vi "EnsaioJigaAutomatizado.vi"() -> ()   [LabVIEW 2025]
uses:
  Estados_Ensaio.ctl
  <vilib>/DAQmx/create/channels.llb/DAQmx Create Channel (DO-Digital Output).vi
  <vilib>/DAQmx/write.llb/DAQmx Write (Digital 1D Bool 1Chan 1Samp).vi
  <vilib>/Utility/file.llb/Write Delimited Spreadsheet (DBL).vi
panel:
  out "Tempo Decorrido (Motor) (s) 2":dbl
  in  "Braco Resistor - 0.68//0.68 2":bool
  in  "Braco Resistor -  0.47//0.47 2":bool
  in  "Braco Resistor - 0.47 2":bool
  in  "Braco Resistor - 1 MOSFET 2":bool
  out "error out 2":errorcluster
  out "Motor  Desligado":i32
  out "Motor Ligado":i32
  in  "module path":path
  in  "Iniciar":bool
  out "Estado Atual":string
  in  "ABORTAR ENSAIO":bool
  out "Tempo Decorrido (Entre braços) (s)":dbl
  out "Tempo Decorrido (Pré-Carga) (s)":dbl
  out "Ativado Braço 7":bool
  out "Pré - Carga Braço 7":bool
  out "Ativado Braço 6":bool
  out "Pré - Carga Braço 6":bool
  out "Ativado Braço 5":bool
  out "Pré - Carga Braço 5":bool
  out "Ativado Braço 4":bool
  out "Pré - Carga Braço 4":bool
  out "Ativado Braço 3":bool
  out "Pré - Carga Braço 3":bool
  out "Ativado Braço  2":bool
  out "Pré - Carga Braço 2":bool
  out "Ativado Braço 1":bool
  out "Pré - Carga Braço 1":bool
  out "Ensaio Iniciado":bool
  in  "Parada while":bool
  in  "Tempo de desligamento entre braços (s)":dbl
  in  "Tempo de pré-carga (s)":dbl
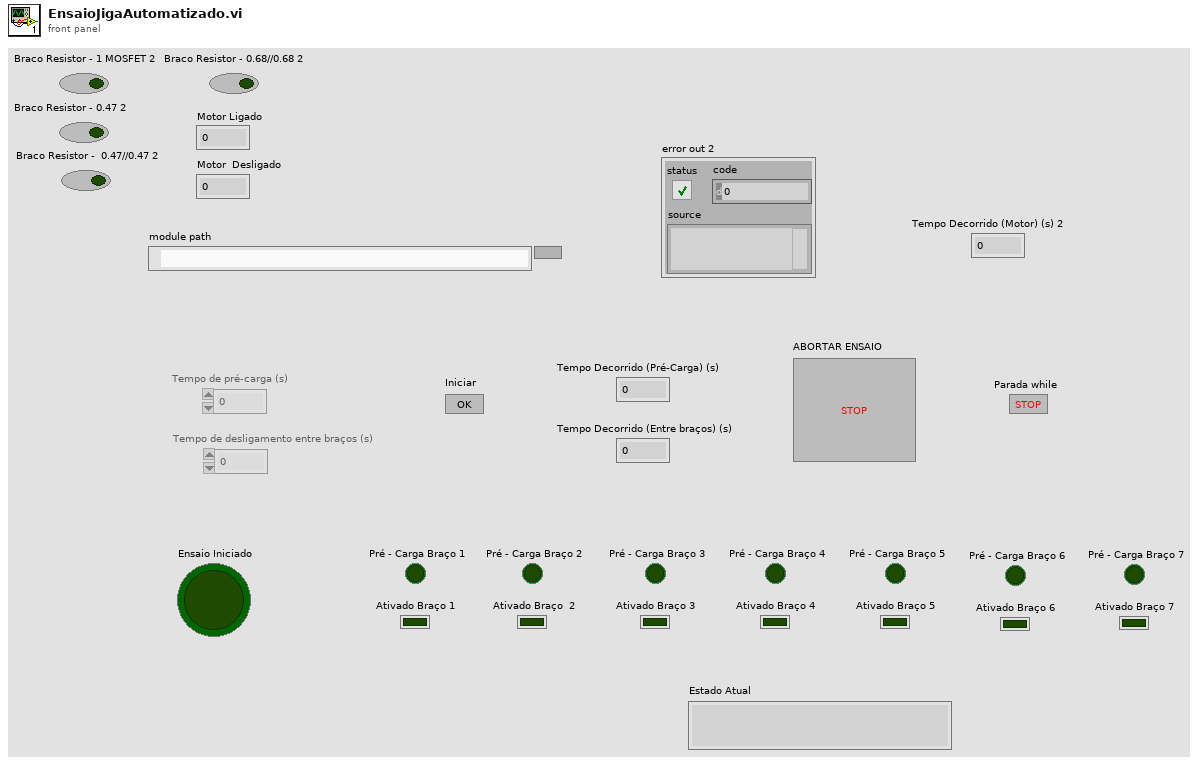
[diagram p1: front panel]
types:
  T1 = typedef "Estados_Ensaio.ctl" = enum16{"Idle", "AtivaPreCarga", "AguardaPreCarga", "AtivaBracosDesativaPreCarga", "DesativaBraco", "Fim", "Abortar", "AtivaBracos", "AguardaAtrasoPreCarga", "ComandoMotor"}
  T2 = enum8{"Enabled", "Disabled", "Disabled and Grayed Out"}
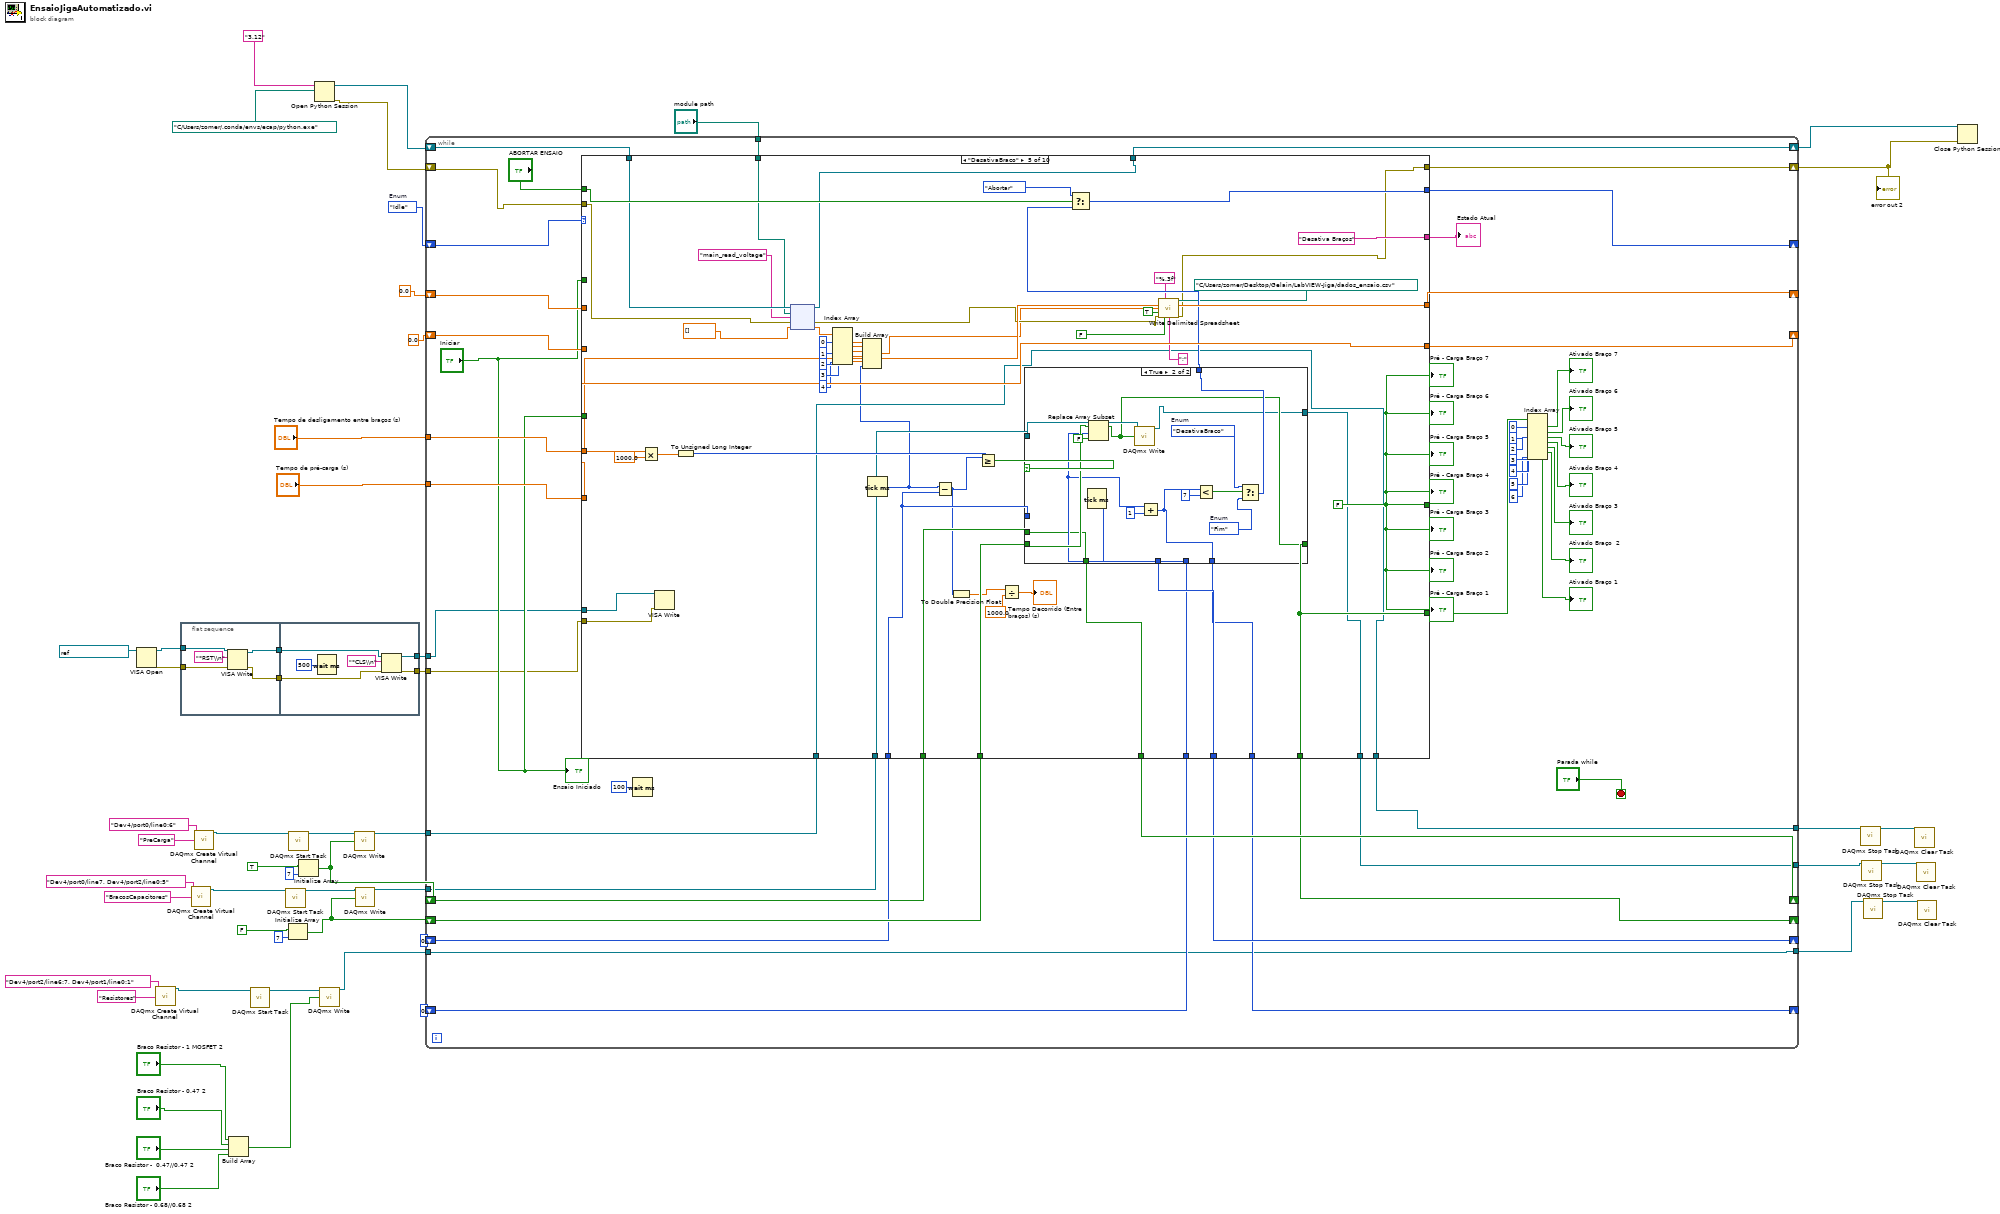
[diagram p0: block diagram]
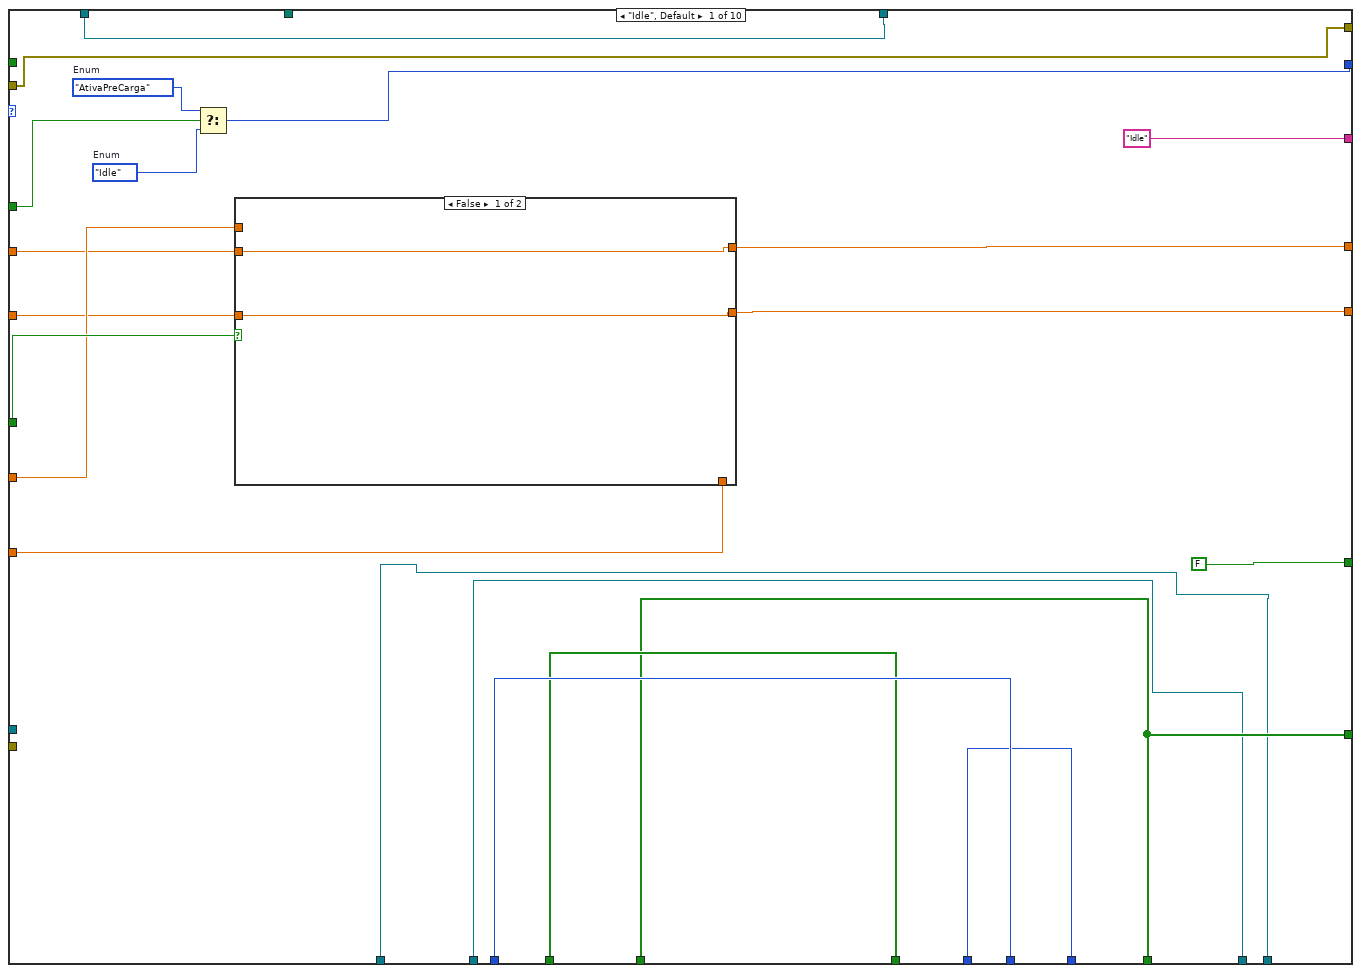
[diagram p2: hidden frame]
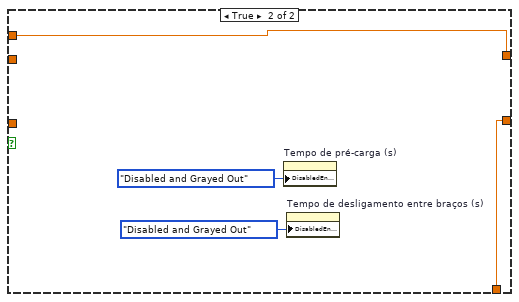
[diagram p3: hidden frame]
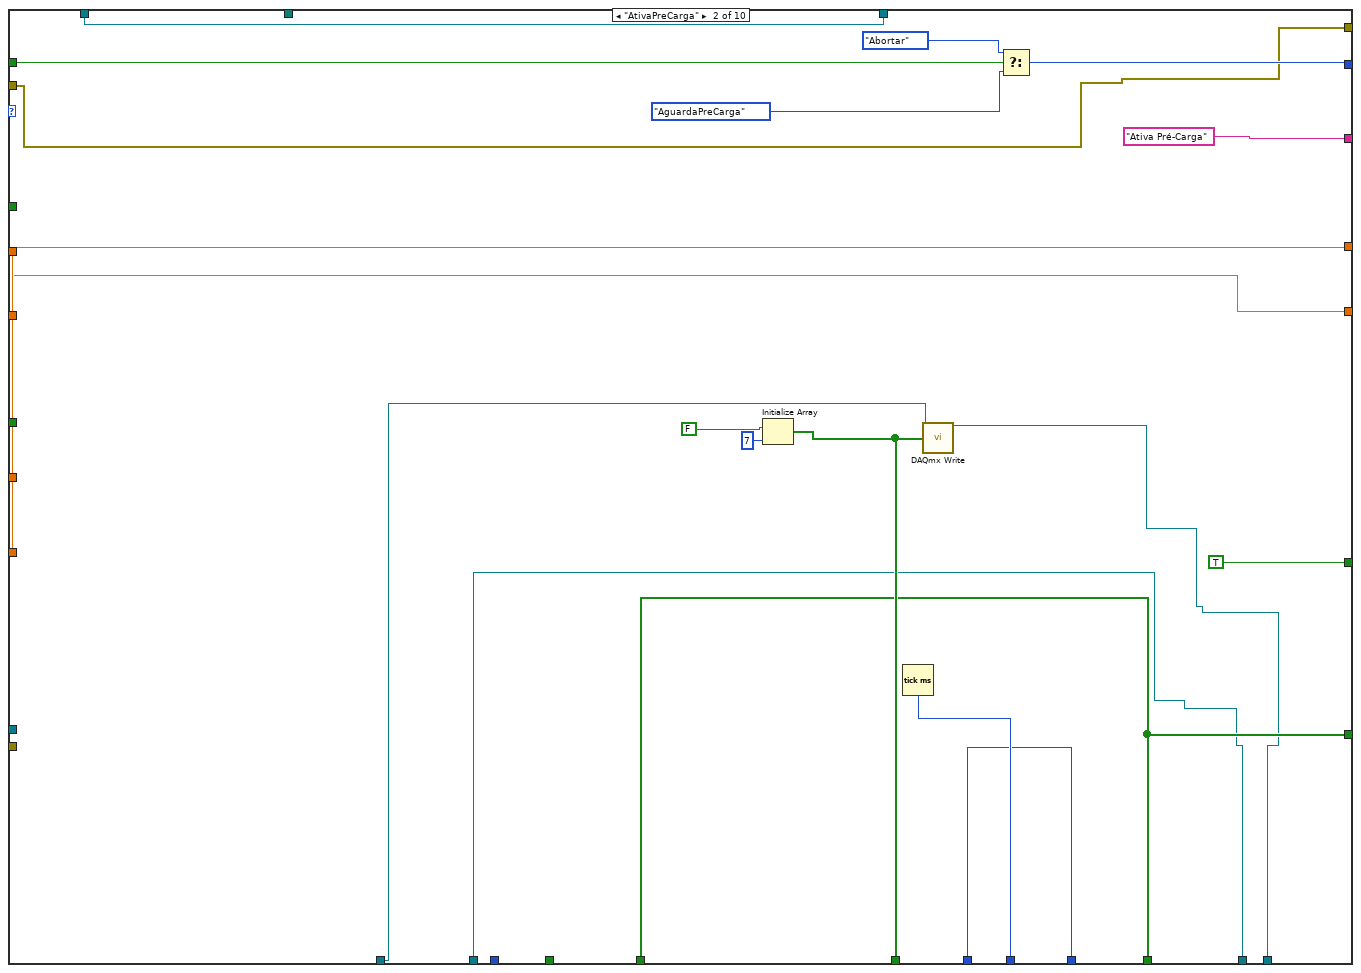
[diagram p4: hidden frame]
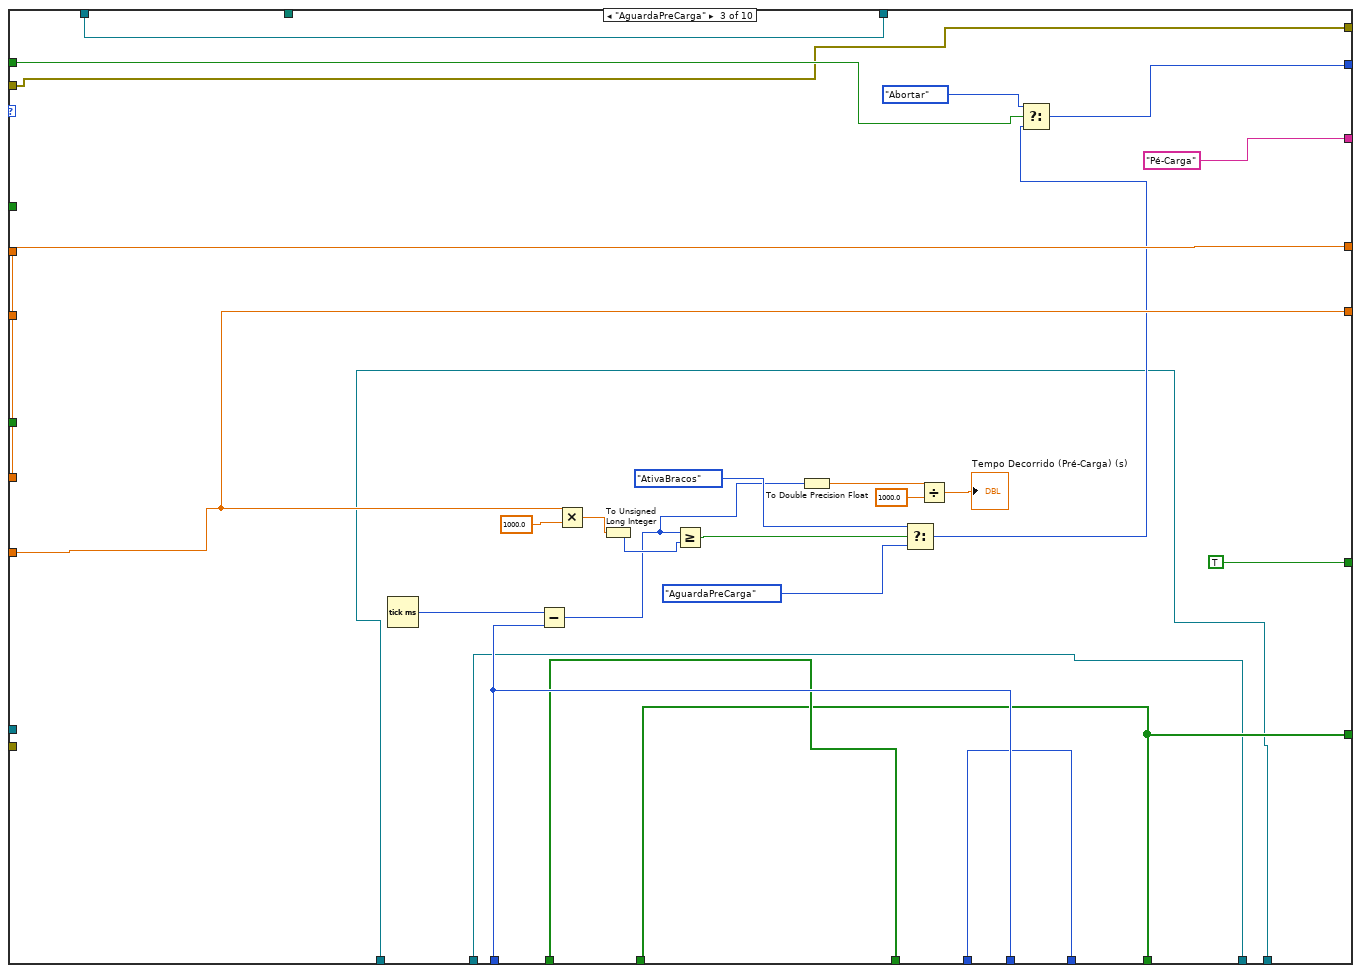
[diagram p5: hidden frame]
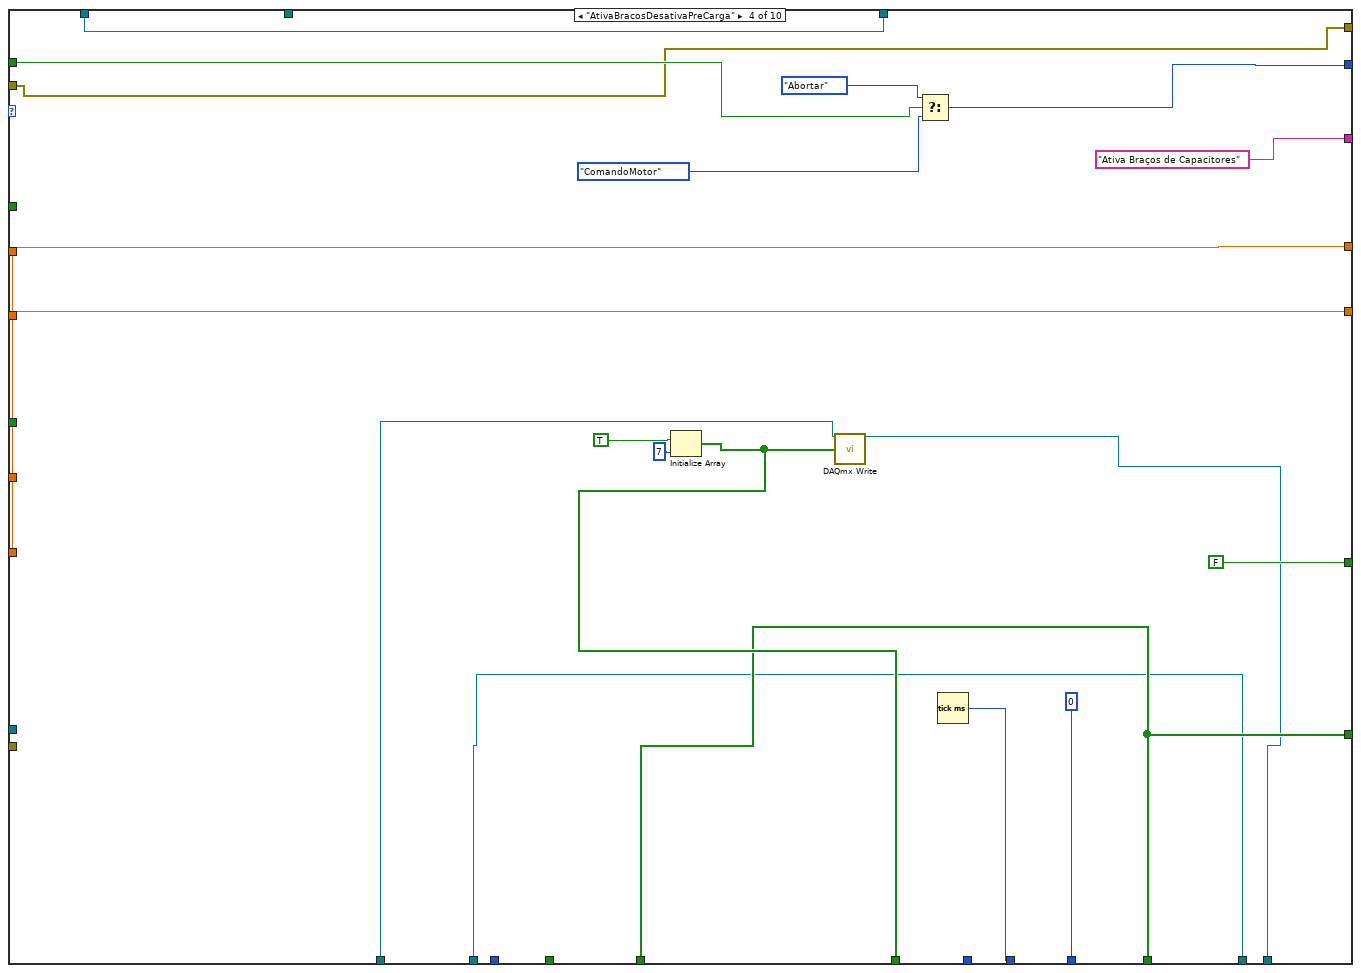
[diagram p6: hidden frame]
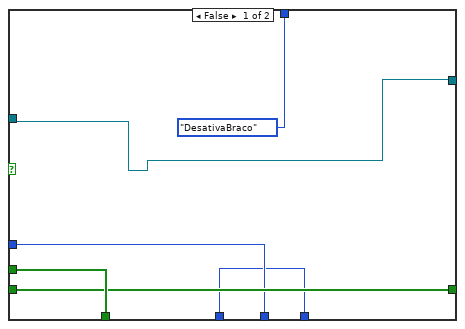
[diagram p7: hidden frame]
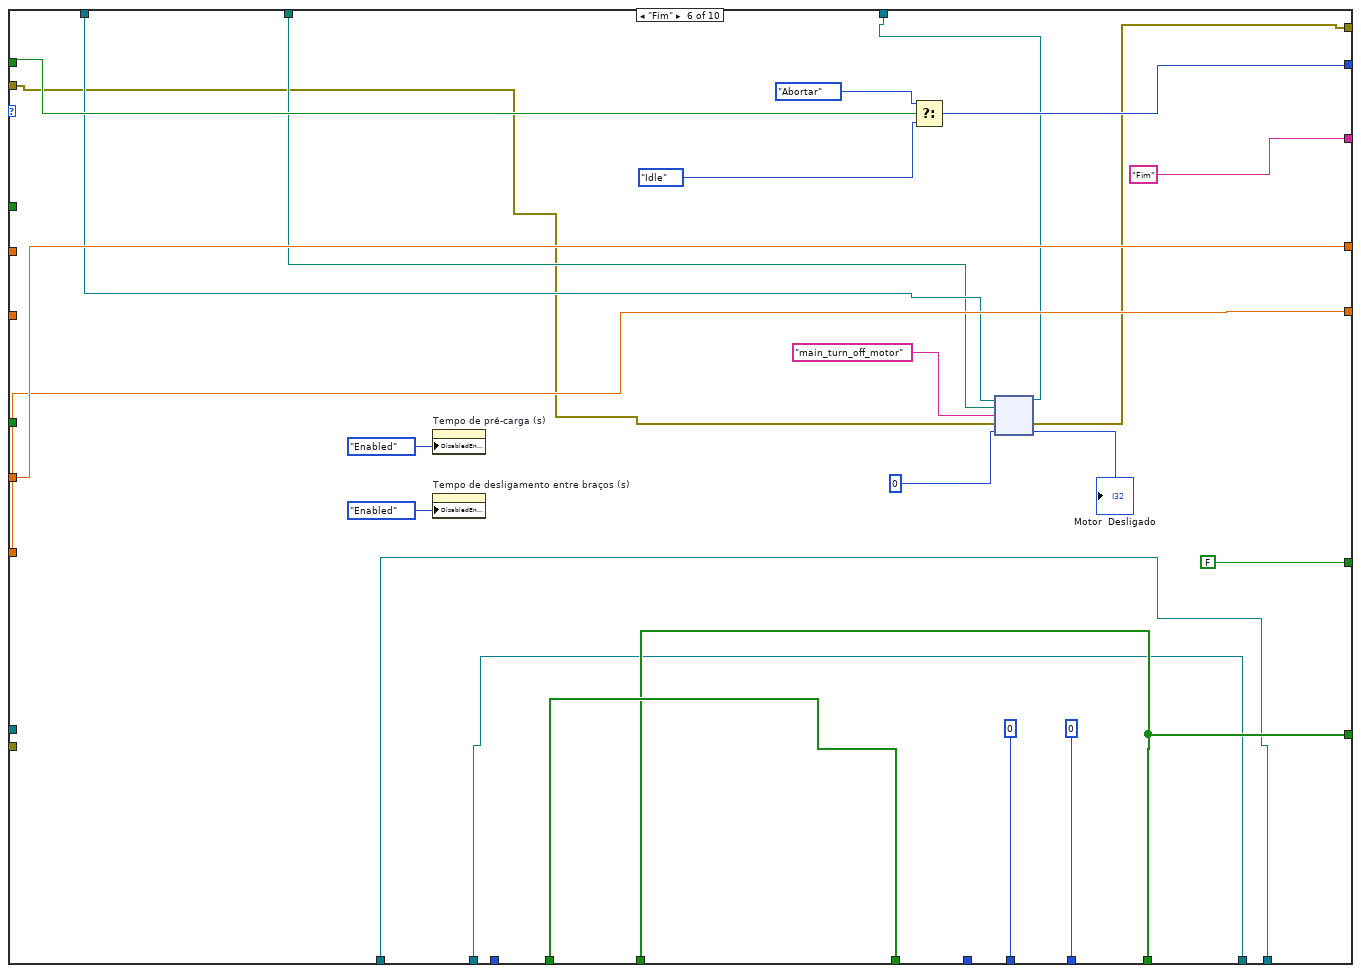
[diagram p8: hidden frame]
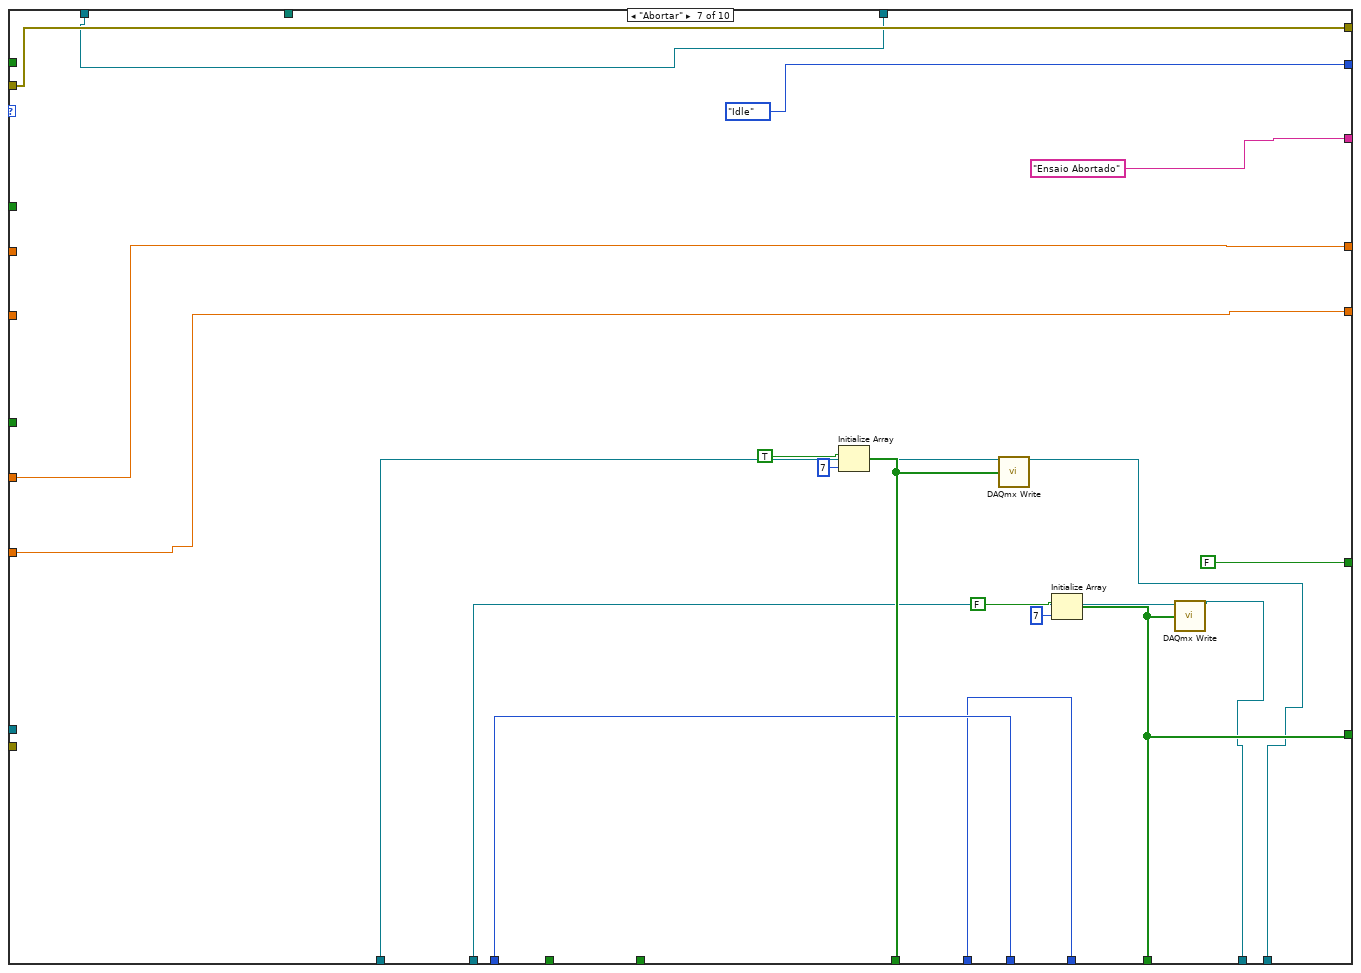
[diagram p9: hidden frame]
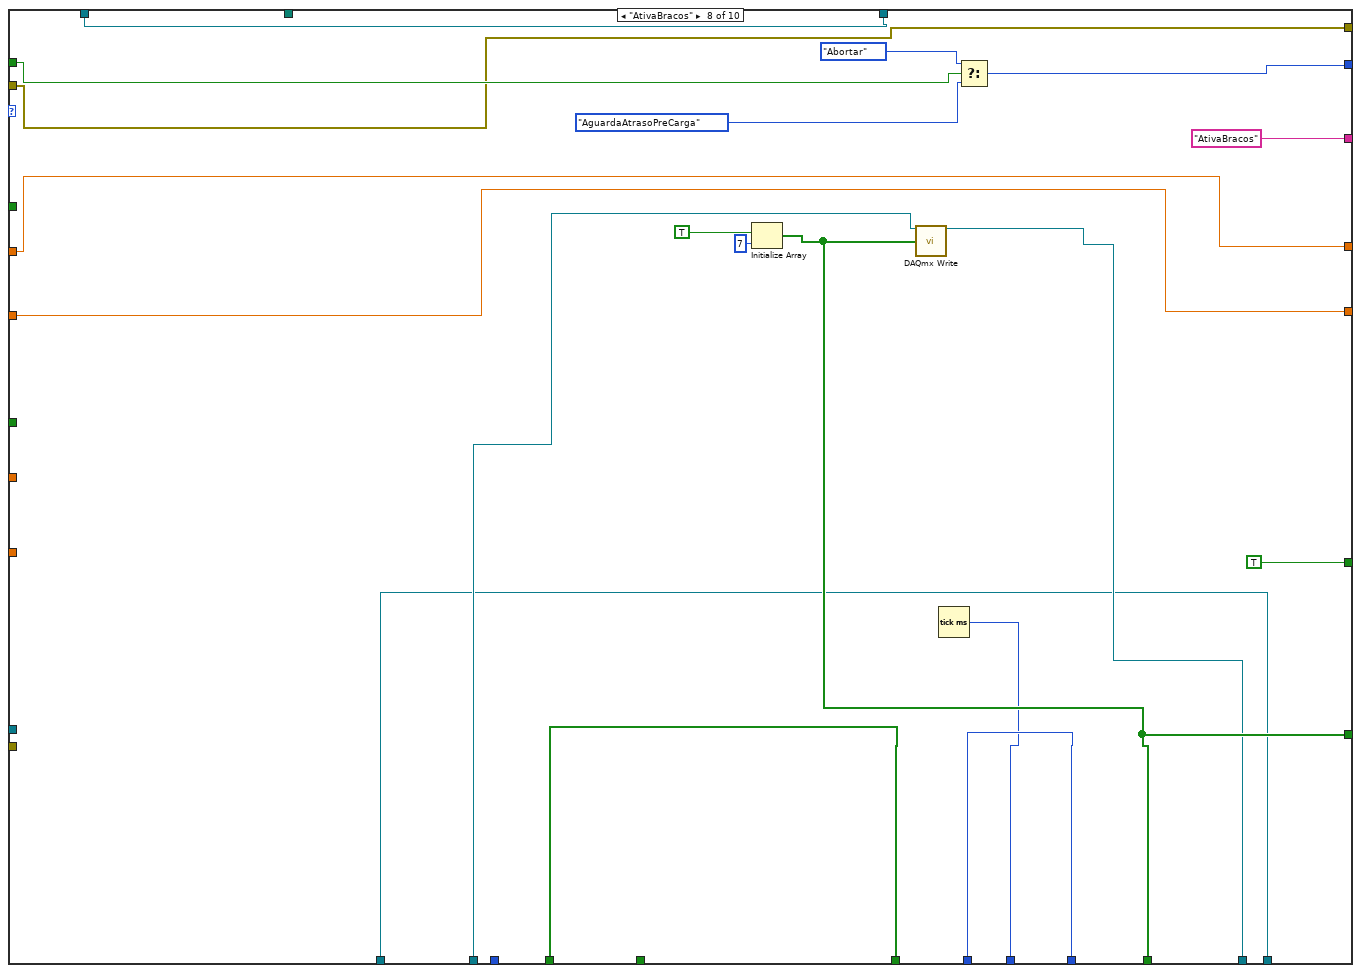
[diagram p10: hidden frame]
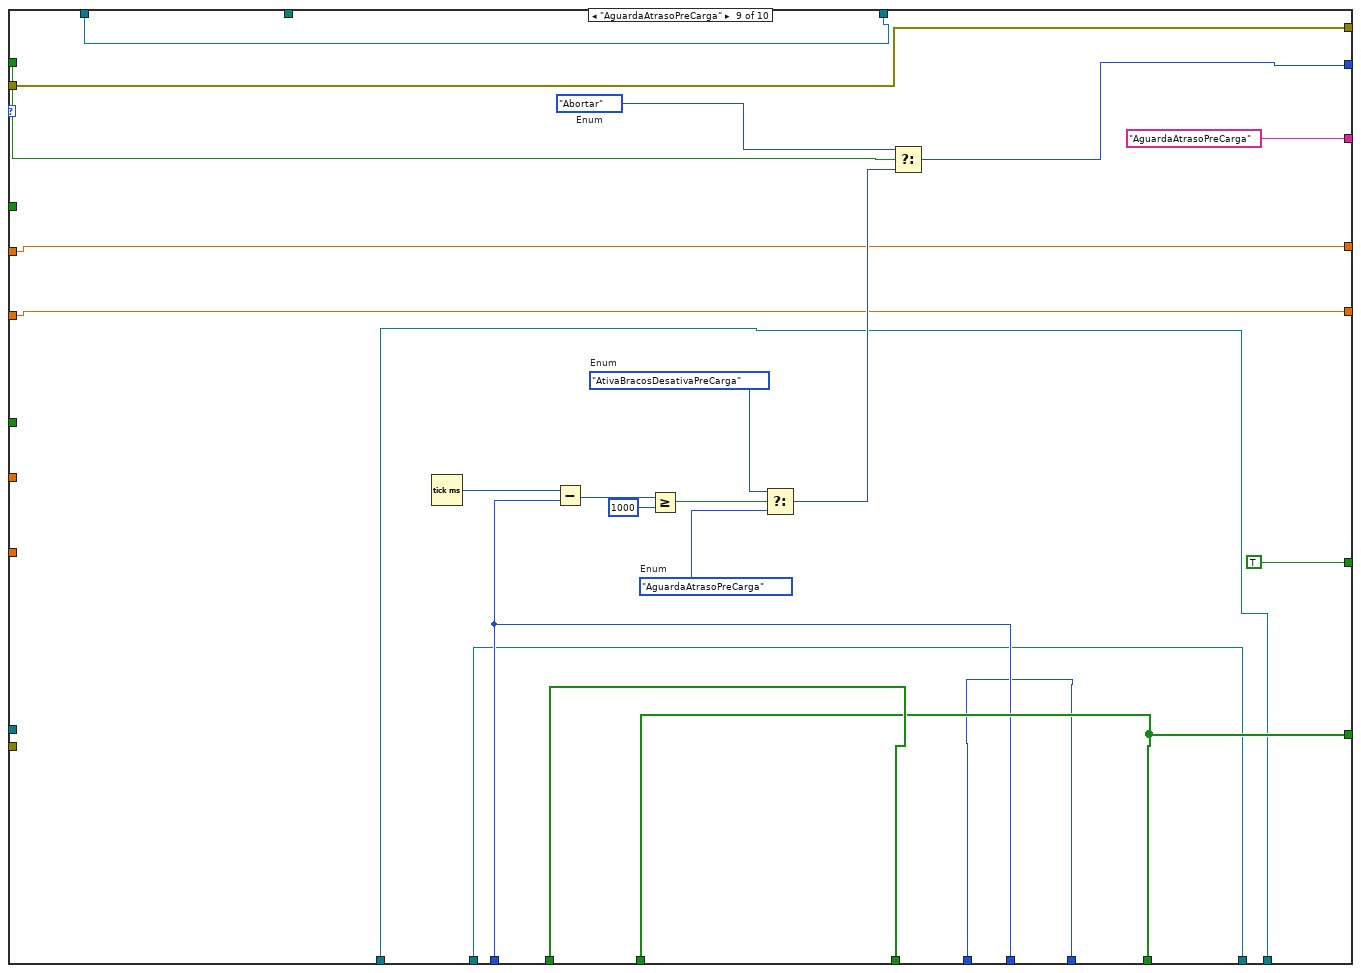
[diagram p11: hidden frame]
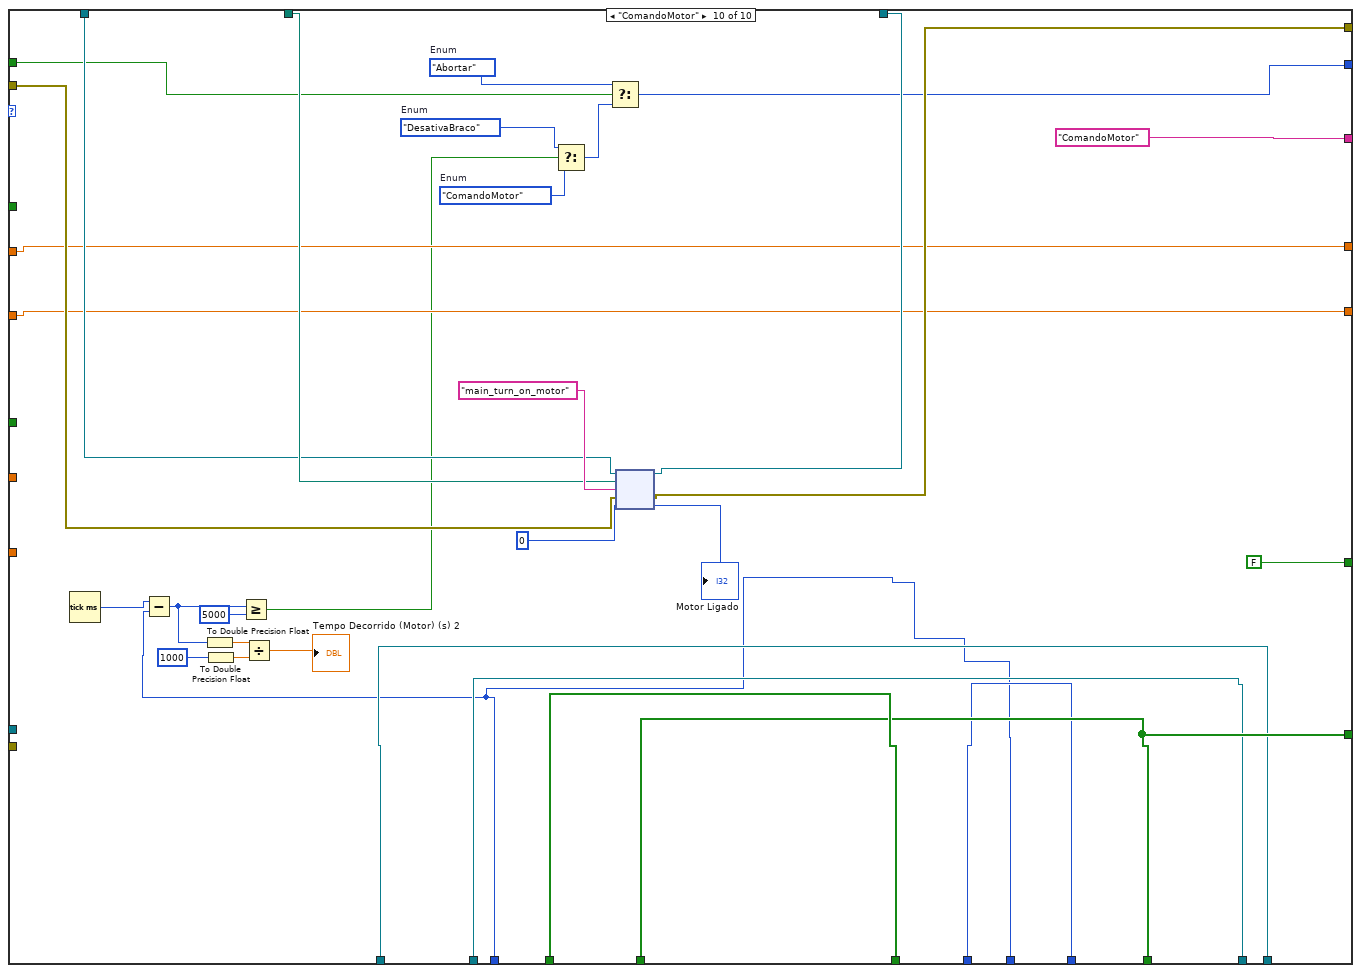
[diagram p12: hidden frame]
diagram:
  w51 = Estados_Ensaio."Idle"  # Enum
  n1 = VISA Open(VISA resource name=refnum<visa-resource-name> "GPIB0::1::INSTR") -> (VISA resource name=w6:refnum<visa-resource-name>, error out=w5:errorcluster)  [unwired: 4 in]
  n2 = call-poly <vilib>:"DAQmx Create Virtual Channel.vi"("lines"=tag "Dev4/port2/line6:7, Dev4/port1/line0:1", "name to assign"="Resistores") -> ("task out"=w17:refnum<k21>)  [unwired: 12 in, 1 out]
  n3 = flat-sequence {
    tunnel: w6 -> [w57]
    tunnel: w5 -> [w56]
    tunnel: [w55] -> w4
    tunnel: [w54] -> w3
    tunnel: w4 -> [w62]
    tunnel: w3 -> [w61]
    tunnel: [w60] -> w2
    tunnel: [w59] -> w1
    frame #0 {
      n4 = VISA Write(VISA resource name=w57, write buffer="*RST\\n", error in (no error)=w56) -> (VISA resource name out=w55:refnum<visa-resource-name>, error out=w54:errorcluster)  [unwired: 1 out]
    }
    frame #1 {
      n5 = Wait (ms)(milliseconds to wait=u32 500) -> ()  [unwired: 1 out]
      n6 = VISA Write(VISA resource name=w62, write buffer="*CLS\\n", error in (no error)=w61) -> (VISA resource name out=w60:refnum<visa-resource-name>, error out=w59:errorcluster)  [unwired: 1 out]
    }
  }
  n7 = call-poly <vilib>:"DAQmx Create Virtual Channel.vi"("lines"=tag "Dev4/port0/line7, Dev4/port2/line0:5", "name to assign"="BracosCapacitores") -> ("task out"=w43:refnum<k21>)  [unwired: 12 in, 1 out]
  n8 = call-poly <vilib>:"DAQmx Create Virtual Channel.vi"("lines"=tag "Dev4/port0/line0:6", "name to assign"="PreCarga") -> ("task out"=w46:refnum<k21>)  [unwired: 12 in, 1 out]
  n9 = Build Array("Braco Resistor - 1 MOSFET 2", "Braco Resistor - 0.47 2", "Braco Resistor -  0.47//0.47 2", "Braco Resistor - 0.68//0.68 2") -> (w11:bool[])
  n10 = call <vilib>:"DAQmx Start Task.vi"("task/channels in"=w17) -> ("task out"=w16:refnum<k21>)  [unwired: 13 in, 1 out]
  n11 = call <vilib>:"DAQmx Start Task.vi"("task/channels in"=w43) -> ("task out"=w39:refnum<k21>)  [unwired: 13 in, 1 out]
  n12 = Initialize Array(FALSE, 7 ("dimension size")) -> (w35:bool[])
  n13 = call <vilib>:"DAQmx Start Task.vi"("task/channels in"=w46) -> ("task out"=w42:refnum<k21>)  [unwired: 13 in, 1 out]
  n14 = Initialize Array(TRUE, 7 ("dimension size")) -> (w34:bool[])
  n15 = Open Python Session(python version="3.12" ("Python version"), python path=path "C:/Users/zomer/.conda/envs/ecap/python.exe" ("Python path")) -> (session out=w27:refnum<k35>, error out=w26:errorcluster)  [unwired: 1 in]
  n16 = call-poly <vilib>:"DAQmx Write.vi"("task/channels in"=w16, "data"=w11) -> ("task out"=w8:refnum<k21>)  [unwired: 11 in, 2 out]
  n17 = call-poly <vilib>:"DAQmx Write.vi"("task/channels in"=w42, "data"=w34) -> ("task out"=w36:refnum<k21>)  [unwired: 11 in, 2 out]
  n18 = call-poly <vilib>:"DAQmx Write.vi"("task/channels in"=w39, "data"=w35) -> ("task out"=w32:refnum<k21>)  [unwired: 11 in, 2 out]
  n19 = while {
    shift-right: [w112] -> _
    shift-left: 0.0 ("Tempo de desligamento entre braços (s)") -> [w107]
    shift-right: [w111] -> _
    shift-left: 0.0 ("Tempo de pré-carga (s)") -> [w106]
    shift-right: [w80] -> _
    shift-left: w51 -> [w79]
    tunnel: "Tempo de desligamento entre braços (s)" -> [w109]
    tunnel: "Tempo de pré-carga (s)" -> [w108]
    shift-right: [w105] -> _
    shift-left: w34 -> [w99]
    shift-right: [w103] -> _
    shift-left: w35 -> [w102]
    shift-right: [w101] -> _
    shift-left: u32 0 ("millisecond timer value") -> [w100]
    tunnel: w36 -> [w104]
    tunnel: w32 -> [w98]
    shift-right: [w97] -> _
    shift-left: 0 -> [w96]
    tunnel: "module path" -> [w75]
    shift-right: [w73] -> w25
    shift-left: w27 -> [w74]
    shift-right: [w71] -> w24
    shift-left: w26 -> [w72]
    tunnel: [w69] -> w23
    tunnel: [w68] -> w20
    tunnel: [w67] -> w9
    tunnel: w8 -> [w67]
    tunnel: w2 -> [w66]
    tunnel: w1 -> [w65]
    stop <- "Parada while" stop-if-true
    n20 = case shown="\"DesativaBraco\"" w79 {
      tunnel: [w130 w148 w167 w193 w237 w294 Estados_Ensaio."Idle" ("Enum") w330 w356 w376] -> w80
      tunnel: "Iniciar" -> [w131 _ _ _ _ _ _ _ _ _]
      tunnel: "Iniciar" -> [w134 _ _ _ _ _ _ _ _ _]
      tunnel: [w133 w154 w186 w205 w241 w305 w323 w336 w354 w386] -> w112
      tunnel: [w132 w153 w178 w204 w260 w304 w322 w335 w353 w385] -> w111
      tunnel: [w120 w151 w174 w191 w246 w297 w314 w340 w350 w382] -> w95
      tunnel: [FALSE ("Pré - Carga Braço 4") TRUE ("Pré - Carga Braço 4") TRUE ("Pré - Carga Braço 4") FALSE ("Pré - Carga Braço 4") FALSE ("Pré - Carga Braço 4") FALSE ("Pré - Carga Braço 4") FALSE ("Pré - Carga Braço 4") TRUE ("Pré - Carga Braço 4") TRUE ("Pré - Carga Braço 4") FALSE ("Pré - Carga Braço 4")] -> w110
      tunnel: w109 -> [w126 w154 w186 w205 w241 w305 w323 _ _ _]
      tunnel: w108 -> [w125 w153 w178 w204 w260 w304 w322 _ _ _]
      tunnel: w107 -> [w124 _ _ _ _ _ _ w336 w354 w386]
      tunnel: w106 -> [w123 _ _ _ _ _ _ w335 w353 w385]
      tunnel: [w121 w157 w177 w200 w255 w298 w318 w338 w351 w383] -> w105
      tunnel: w104 -> [w115 w156 w161 w199 w222 w283 w317 w325 w344 w379]
      tunnel: [w120 w151 w174 w191 w246 w297 w314 w340 w350 w382] -> w103
      tunnel: w102 -> [w120 w151 w174 w191 w248 w297 _ _ w350 w382]
      tunnel: [w122 w152 w179 w198 w253 u32 0 ("millisecond timer value") w312 w329 w349 w366] -> w101
      tunnel: w100 -> [w122 _ w179 _ w252 _ w312 _ w349 w366]
      tunnel: w99 -> [w121 _ w177 _ w254 w298 _ w338 w351 w383]
      tunnel: w98 -> [w114 w141 w160 w187 w249 w282 w313 w341 w345 w380]
      tunnel: [w119 w150 w173 0 w251 0 w311 w337 w348 w381] -> w97
      tunnel: w96 -> [w119 w150 w173 _ w250 _ w311 w337 w348 w381]
      tunnel: "ABORTAR ENSAIO" -> [_ w147 w165 w194 w238 w293 _ w331 w358 w388]
      tunnel: ["Idle" "Ativa Pré-Carga" "Pé-Carga" "Ativa Braços de Capacitores" "Desativa Braços" "Fim" "Ensaio Abortado" "AtivaBracos" "AguardaAtrasoPreCarga" "ComandoMotor"] -> w77
      tunnel: w75 -> [_ _ _ _ w233 w287 _ _ _ w393]
      tunnel: w74 -> [w117 w144 w163 w190 w235 w288 w308 w328 w347 w392]
      tunnel: [w117 w144 w163 w190 w232 w285 w308 w328 w347 w391] -> w73
      tunnel: w72 -> [w116 w143 w162 w189 w231 w286 w309 w327 w346 w390]
      tunnel: [w116 w143 w162 w189 w224 w284 w309 w327 w346 w389] -> w71
      tunnel: [w115 w142 w161 w188 w222 w283 w307 w325 w344 w379] -> w69
      tunnel: [w114 w141 w160 w187 w223 w282 w306 w326 w345 w380] -> w68
      tunnel: w66 -> [_ _ _ _ w207 _ _ _ _ _]
      tunnel: w65 -> [_ _ _ _ w206 _ _ _ _ _]
      frame "Idle", Default {
        w128 = Estados_Ensaio."Idle"  # Enum
        w129 = Estados_Ensaio."AtivaPreCarga"  # Enum
        n21 = Select(t=w129, s=w131, f=w128) -> (s? t:f=w130:T1)
        n22 = case shown="False" w134 {
          tunnel: [w136 w138] -> w133
          tunnel: [w135 w137] -> w132
          tunnel: w126 -> [_ w138]
          tunnel: w125 -> [_ w137]
          tunnel: w124 -> [w136 _]
          tunnel: w123 -> [w135 _]
          frame False {
          }
          frame True {
            n23 = property on="Tempo de pré-carga (s)" class="DigNum (strict)"("DisabledEnum"=T2."Disabled and Grayed Out" ("Disabled")) -> ()  [unwired: 2 in, 2 out]
            n24 = property on="Tempo de desligamento entre braços (s)" class="DigNum (strict)"("DisabledEnum"=T2."Disabled and Grayed Out" ("Disabled")) -> ()  [unwired: 2 in, 2 out]
          }
        }
      }
      frame "AtivaPreCarga" {
        n25 = Initialize Array(FALSE, 7 ("dimension size")) -> (w157:bool[])
        n26 = Tick Count (ms)() -> (millisecond timer value=w152:u32)
        n27 = call-poly <vilib>:"DAQmx Write.vi"("task/channels in"=w156, "data"=w157) -> ("task out"=w142:refnum<k21>)  [unwired: 11 in, 2 out]
        n28 = Select(t=Estados_Ensaio."Abortar" ("Enum"), s=w147, f=Estados_Ensaio."AguardaPreCarga" ("Enum")) -> (s? t:f=w148:T1)
      }
      frame "AguardaPreCarga" {
        n29 = Tick Count (ms)() -> (millisecond timer value=w184:u32)
        n30 = Subtract(x=w184, y=w179) -> (x-y=w171:u32)
        n31 = Multiply(x=w178, y=1000.0) -> (x*y=w176:dbl)
        n32 = To Unsigned Long Integer(number=w176) -> (unsigned 32bit integer=w175:u32)
        n33 = Greater Or Equal?(x=w171, y=w175) -> (x >= y?=w182:bool)
        n34 = To Double Precision Float(number=w171) -> (double precision float=w170:dbl)
        n35 = Select(t=Estados_Ensaio."AtivaBracos" ("Enum"), s=w182, f=Estados_Ensaio."AguardaPreCarga" ("Enum")) -> (s? t:f=w166:T1)
        n36 = Divide(x=w170, y=1000.0) -> (x/y=→"Tempo Decorrido (Pré-Carga) (s)":dbl)
        n37 = Select(t=Estados_Ensaio."Abortar" ("Enum"), s=w165, f=w166) -> (s? t:f=w167:T1)
      }
      frame "AtivaBracosDesativaPreCarga" {
        n38 = Initialize Array(TRUE, 7 ("dimension size")) -> (w200:bool[])
        n39 = call-poly <vilib>:"DAQmx Write.vi"("task/channels in"=w199, "data"=w200) -> ("task out"=w188:refnum<k21>)  [unwired: 11 in, 2 out]
        n40 = Select(t=Estados_Ensaio."Abortar" ("Enum"), s=w194, f=Estados_Ensaio."ComandoMotor" ("Enum")) -> (s? t:f=w193:T1)
        n41 = Tick Count (ms)() -> (millisecond timer value=w198:u32)
      }
      frame "DesativaBraco" {
        n42 = Multiply(x=w241, y=1000.0) -> (x*y=w258:dbl)
        n43 = VISA Write(VISA resource name=w207, error in (no error)=w206) -> ()  [unwired: 1 in, 3 out]
        n44 = To Unsigned Long Integer(number=w258) -> (unsigned 32bit integer=w257:u32)
        n45 = node(w235, w233, "main_read_voltage" ("function name"), w231, dbl[] []) -> (w232:refnum<k35>, w225:errorcluster, w220:dbl[])  [unwired: 2 out]
        n46 = Index Array(array=w220, index #1=0 ("index"), index #2=1 ("index"), index #3=2 ("index"), index #4=3 ("index"), index #5=4 ("index")) -> (element #1=w214:dbl, element #2=w213:dbl, element #3=w212:dbl, element #4=w211:dbl, element #5=w210:dbl)
        n47 = Tick Count (ms)() -> (millisecond timer value=w208:u32)
        n48 = Build Array(w214, w213, w212, w211, w210, w208) -> (w209:dbl[])
        n49 = Subtract(x=w208, y=w252) -> (x-y=w245:u32)
        n50 = To Double Precision Float(number=w245) -> (double precision float=w243:dbl)
        n51 = Greater Or Equal?(x=w245, y=w257) -> (x >= y?=w256:bool)
        n52 = Divide(x=w243, y=1000.0) -> (x/y=→"Tempo Decorrido (Entre braços) (s)":dbl)
        n53 = case shown="True" w256 {
          tunnel: [w266 w268] -> w255
          tunnel: w254 -> [w266 w268]
          tunnel: [w265 w269] -> w246
          tunnel: w248 -> [w265 w281]
          tunnel: [w264 w278] -> w253
          tunnel: w252 -> [w264 _]
          tunnel: [w263 w275] -> w251
          tunnel: w250 -> [w263 w277]
          tunnel: [Estados_Ensaio."DesativaBraco" ("Enum") w270] -> w239
          tunnel: w249 -> [w261 w279]
          tunnel: [w261 w267] -> w223
          frame False {
          }
          frame True {
            w271 = Estados_Ensaio."Fim"  # Enum
            w272 = Estados_Ensaio."DesativaBraco"  # Enum
            n54 = Tick Count (ms)() -> (millisecond timer value=w278:u32)
            n55 = Replace Array Subset(array=w281, new element=FALSE ("new element/subarray"), index=w277) -> (w269:bool[])
            n56 = call-poly <vilib>:"DAQmx Write.vi"("task/channels in"=w279, "data"=w269) -> ("task out"=w267:refnum<k21>)  [unwired: 11 in, 2 out]
            n57 = Add(x=w277, y=1) -> (x+y=w275:i32)
            n58 = Less?(x=w275, y=7) -> (x < y?=w273:bool)
            n59 = Select(t=w272, s=w273, f=w271) -> (s? t:f=w270:T1)
          }
        }
        n60 = Select(t=Estados_Ensaio."Abortar" ("Enum"), s=w238, f=w239) -> (s? t:f=w237:T1)
        n61 = call-poly <vilib>:"Write Delimited Spreadsheet.vi"("file path (dialog if empty)"=path "C:/Users/zomer/Desktop/Gelain/LabVIEW-Jiga/dados_ensaio.csv", "format (%.3f)"="%.3f", "1D data"=w209, "append to file? (new file:F)"=TRUE, "error in (no error)"=w225, "transpose? (no:F)"=FALSE, "delimiter (\\t)"=";" ("delimiter (\\t)")) -> ("error out"=w224:errorcluster)  [unwired: 7 in, 1 out]
      }
      frame "Fim" {
        n62 = property on="Tempo de pré-carga (s)" class="DigNum (strict)"("DisabledEnum"=T2."Enabled" ("Disabled")) -> ()  [unwired: 2 in, 2 out]
        n63 = property on="Tempo de desligamento entre braços (s)" class="DigNum (strict)"("DisabledEnum"=T2."Enabled" ("Disabled")) -> ()  [unwired: 2 in, 2 out]
        n64 = Select(t=Estados_Ensaio."Abortar" ("Enum"), s=w293, f=Estados_Ensaio."Idle" ("Enum")) -> (s? t:f=w294:T1)
        n65 = node(w288, w287, "main_turn_off_motor" ("function name"), w286, 0) -> (w285:refnum<k35>, w284:errorcluster, →"Motor  Desligado":i32)  [unwired: 2 out]
      }
      frame "Abortar" {
        n66 = Initialize Array(TRUE, 7 ("dimension size")) -> (w318:bool[])
        n67 = call-poly <vilib>:"DAQmx Write.vi"("task/channels in"=w317, "data"=w318) -> ("task out"=w307:refnum<k21>)  [unwired: 11 in, 2 out]
        n68 = Initialize Array(FALSE, 7 ("dimension size")) -> (w314:bool[])
        n69 = call-poly <vilib>:"DAQmx Write.vi"("task/channels in"=w313, "data"=w314) -> ("task out"=w306:refnum<k21>)  [unwired: 11 in, 2 out]
      }
      frame "AtivaBracos" {
        n70 = Initialize Array(TRUE, 7 ("dimension size")) -> (w340:bool[])
        n71 = call-poly <vilib>:"DAQmx Write.vi"("task/channels in"=w341, "data"=w340) -> ("task out"=w326:refnum<k21>)  [unwired: 11 in, 2 out]
        n72 = Tick Count (ms)() -> (millisecond timer value=w329:u32)
        n73 = Select(t=Estados_Ensaio."Abortar" ("Enum"), s=w331, f=Estados_Ensaio."AguardaAtrasoPreCarga" ("Enum")) -> (s? t:f=w330:T1)
      }
      frame "AguardaAtrasoPreCarga" {
        w357 = Estados_Ensaio."Abortar"  # Enum
        w360 = Estados_Ensaio."AtivaBracosDesativaPreCarga"  # Enum
        w361 = Estados_Ensaio."AguardaAtrasoPreCarga"  # Enum
        n74 = Tick Count (ms)() -> (millisecond timer value=w365:u32)
        n75 = Subtract(x=w365, y=w349) -> (x-y=w364:u32)
        n76 = Greater Or Equal?(x=w364, y=u32 1000) -> (x >= y?=w362:bool)
        n77 = Select(t=w360, s=w362, f=w361) -> (s? t:f=w359:T1)
        n78 = Select(t=w357, s=w358, f=w359) -> (s? t:f=w356:T1)
      }
      frame "ComandoMotor" {
        w374 = Estados_Ensaio."DesativaBraco"  # Enum
        w375 = Estados_Ensaio."ComandoMotor"  # Enum
        w387 = Estados_Ensaio."Abortar"  # Enum
        n79 = Tick Count (ms)() -> (millisecond timer value=w378:u32)
        n80 = Subtract(x=w378, y=w366) -> (x-y=w370:u32)
        n81 = To Double Precision Float(number=w370) -> (double precision float=w371:dbl)
        n82 = To Double Precision Float(number=u32 1000 ("y")) -> (double precision float=w368:dbl)
        n83 = Greater Or Equal?(x=w370, y=u32 5000) -> (x >= y?=w373:bool)
        n84 = Divide(x=w371, y=w368) -> (x/y=→"Tempo Decorrido (Motor) (s) 2":dbl)
        n85 = Select(t=w374, s=w373, f=w375) -> (s? t:f=w377:T1)
        n86 = Select(t=w387, s=w388, f=w377) -> (s? t:f=w376:T1)
        n87 = node(w392, w393, "main_turn_on_motor" ("function name"), w390, 0) -> (w391:refnum<k35>, w389:errorcluster, →"Motor Ligado":i32)  [unwired: 2 out]
      }
    }
    "Pré - Carga Braço 7" <- w110
    "Pré - Carga Braço 6" <- w110
    "Pré - Carga Braço 5" <- w110
    "Pré - Carga Braço 4" <- w110
    "Pré - Carga Braço 3" <- w110
    "Pré - Carga Braço 2" <- w110
    "Pré - Carga Braço 1" <- w110
    "Estado Atual" <- w77
    n88 = Wait (ms)(milliseconds to wait=u32 100) -> ()  [unwired: 1 out]
    n89 = Index Array(array=w95, index #1=0 ("index"), index #2=1 ("index"), index #3=2 ("index"), index #4=3 ("index"), index #5=4 ("index"), index #6=5 ("index"), index #7=6 ("index")) -> (element #1=→"Ativado Braço 7":bool, element #2=→"Ativado Braço 6":bool, element #3=→"Ativado Braço 5":bool, element #4=→"Ativado Braço 4":bool, element #5=→"Ativado Braço 3":bool, element #6=→"Ativado Braço  2":bool, element #7=→"Ativado Braço 1":bool)
    "Ensaio Iniciado" <- "Iniciar"
  }
  "error out 2" <- w24
  n90 = call <vilib>:"DAQmx Stop Task.vi"("task/channels in"=w23) -> ("task out"=w22:refnum<k21>)  [unwired: 13 in, 1 out]
  n91 = call <vilib>:"DAQmx Stop Task.vi"("task/channels in"=w20) -> ("task out"=w21:refnum<k21>)  [unwired: 13 in, 1 out]
  n92 = call <vilib>:"DAQmx Stop Task.vi"("task/channels in"=w9) -> ("task out"=w10:refnum<k21>)  [unwired: 13 in, 1 out]
  n93 = call <vilib>:"DAQmx Clear Task.vi"("task in"=w22) -> ()  [unwired: 14 in, 1 out]
  n94 = call <vilib>:"DAQmx Clear Task.vi"("task in"=w21) -> ()  [unwired: 14 in, 1 out]
  n95 = call <vilib>:"DAQmx Clear Task.vi"("task in"=w10) -> ()  [unwired: 14 in, 1 out]
  n96 = Close Python Session(session in=w25, error in=w24) -> ()  [unwired: 1 out]
